vi "lv-build.vi"() -> ()   [LabVIEW 2014, in "lv-cli-steps.lvlib"]
uses:
  lv-cli-steps.lvlib
  <vilib>/Utility/error.llb/DialogType.ctl
  <vilib>/AppBuilder/AB_API_Simple/Build (path).vi
  <vilib>/Wiresmith Technology/LabVIEW CLI/CLI Class/CLI.lvclass
  <vilib>/AppBuilder/AB_API_Simple/NI_App_Builder_API.lvlib
panel:
  out "error out":errorcluster
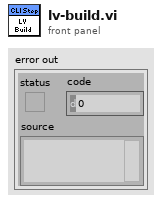
[diagram p1: front panel]
types:
  T1 = typedef "DialogType.ctl" = u16
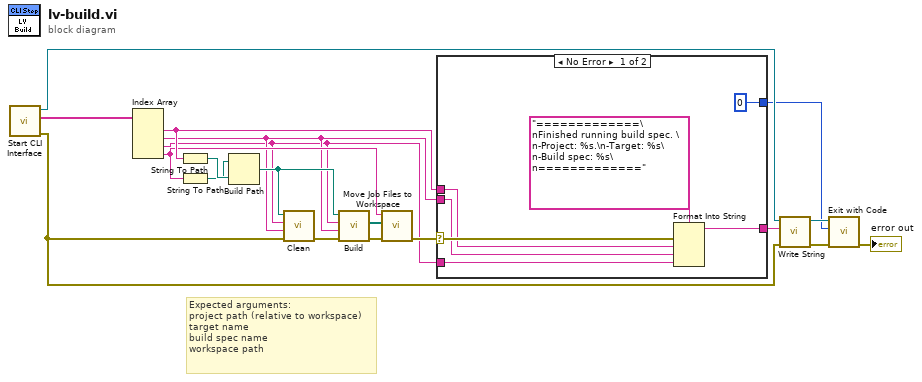
[diagram p0: block diagram]
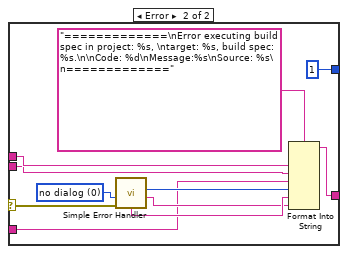
[diagram p2: hidden frame]
diagram:
  # "Expected arguments:\nproject path (relative to workspace)\ntarget name\nbuild spec name\nworkspace path"
  n1 = call <vilib>:"Start CLI Interface.vi"() -> ("error out"=w1:errorcluster, "Custom Parameters"=w19:string[], "CLI out"=w16:refnum<class "CLI.lvclass">)  [unwired: 9 in]
  n2 = Index Array(array=w19) -> (element #1=w18:string, element #2=w3:string, element #3=w2:string, element #4=w4:string)  [unwired: 4 in]
  n3 = String To Path(string=w18) -> (path=w12:path)
  n4 = String To Path(string=w4) -> (path=w11:path)
  n5 = Build Path(base path=w11, name or relative path=w12) -> (appended path=w5:path)
  n6 = call <vilib>:"Clean.vi"("error in (no error)"=w1, "Name of target (My Computer)"=w3, "Name of build specification (if empty: clean all)"=w2, "Path to project"=w5) -> ("error out"=w8:errorcluster)  [unwired: 7 in]
  n7 = call-poly <vilib>:"Build.vi"("error in (no error)"=w8, "Name of target (My Computer)"=w3, "Name of build specification (if empty: build all)"=w2, "Path to project"=w5) -> ("error out"=w7:errorcluster, "Generated files"=w6:path[])  [unwired: 6 in]
  n8 = call "Move Job Files to Workspace.vi"("error in (no error)"=w7, "Generated Files"=w6, "Workspace Path"=w4) -> ("error out"=w10:errorcluster)  [unwired: 8 in]
  n9 = case shown="No Error" w10 {
    selector: w10 -> [w25 w36]
    tunnel: w18 -> [w24 w29]
    tunnel: w3 -> [w23 w28]
    tunnel: [w22 w37] -> w17
    tunnel: [0 ("Exit Code (0)") 1 ("Exit Code (0)")] -> w13
    tunnel: w2 -> [w20 w27]
    frame No Error {
      n10 = Format Into String(format string="=============\nFinished running build spec. \n-Project: %s.\n-Target: %s\n-Build spec: %s\n=============", error in=w25, w24, w23, w20) -> (resulting string=w22:string)  [unwired: 1 in, 1 out]
    }
    frame Error {
      w35 = T1 0 items=["no dialog", "OK message", "continue or stop message", "OK message + warnings", "continue/stop + warnings"] ("type of dialog (OK msg:1)")
      n11 = call <vilib>:"Simple Error Handler.vi"("type of dialog (OK msg:1)"=w35, "error in (no error)"=w36) -> ("code out"=w30:i32, "source out"=w31:string, "message"=w32:string)  [unwired: 3 in, 2 out]
      n12 = Format Into String(format string="=============\nError executing build spec in project: %s, \ntarget: %s, build spec: %s.\n\nCode: %d\nMessage:%s\nSource: %s\n=============", w29, w28, w27, w30, w32, w31) -> (resulting string=w37:string)  [unwired: 2 in, 1 out]
    }
  }
  n13 = call <vilib>:"Write String.vi"("error in (no error)"=w1, "Text to Write"=w17, "CLI in"=w16) -> ("error out"=w15:errorcluster, "CLI out"=w14:refnum<class "CLI.lvclass">)  [unwired: 7 in]
  n14 = call <vilib>:"Exit with Code.vi"("error in (no error)"=w15, "Exit Code (0)"=w13, "CLI in"=w14) -> ("error out"=→"error out":errorcluster)  [unwired: 8 in]
